vi "Get_Shutter_Status.vi"(8 "error in (no error)":errorcluster, 11 ".NET Reference in":refnum<k24>) -> (0 "error out":errorcluster, 2 "status":enum16{"Shutter_Open", "Shutter_Close", ""}(ring), 3 "Reference out":refnum<k24>)   [LabVIEW 2017]
uses:
  C:/Users/Ssantec_Test/Documents/Instrument_DLL_Sample_Labview_20250826_Ver1.5.0_x64/DLL/InstrumentDLL.dll
  DLL/InstrumentDLL.dll
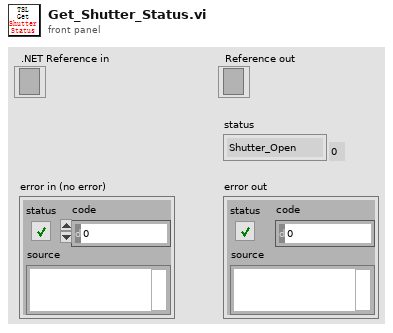
[diagram p1: front panel]
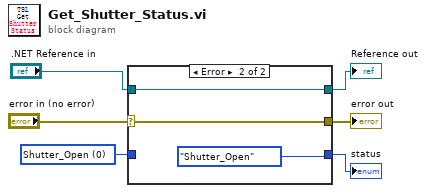
[diagram p0: block diagram]
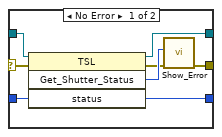
[diagram p2: hidden frame]
diagram:
  w2 = 0 items=["Shutter_Open", "Shutter_Close"] ("status")
  n1 = case shown="Error" "error in (no error)" {
    selector: "error in (no error)" -> [w7 w16]
    tunnel: [w14 enum16{"Shutter_Open", "Shutter_Close", ""}."Shutter_Open" ("status")] -> w6
    tunnel: ".NET Reference in" -> [w13 w17]
    tunnel: [w12 w17] -> w4
    tunnel: [w8 w16] -> w3
    tunnel: w2 -> [w11 _]
    frame No Error {
      n2 = invoke on="调用节点" class="TSL" method="Get_Shutter_Status"(reference=w13, error in=w7, "status"=w11) -> (reference out=w12:refnum<k24>, error out=w9:errorcluster, "Get_Shutter_Status"=w10:i32, "status"=w14:i32)  [unwired: 1 in]
      n3 = call "Show_Error.vi"("error in (no error)"=w9, "Error"=w10) -> ("error out"=w8:errorcluster)  [unwired: 9 in]
    }
    frame Error {
    }
  }
  "Reference out" <- w4
  "error out" <- w3
  "status" <- w6
